vi "ini_file_read_pulse_tx.vi"(8 "error in (no error)":errorcluster, 11 "secnario config":T1={"devicess 2"=["IF_transiver_1", "IF_transiver_2"], "file paths"=[path "C:/Users/PXIe8108_Demo/Documents/CHAIM DATA/chaim/5785_sync_for_elbit/data/pdw_test_file.tdms", path "C:/Users/PXIe8108_Demo/Documents/CHAIM DATA/chaim/5785_sync_for_elbit/data/pdw_test_file.tdms", path "C:/Users/PXIe8108_Demo/Documents/CHAIM DATA/chaim/5785_sync_for_elbit/data/pdw_test_file.tdms", path "C:/Users/PXIe8108_Demo/Documents/CHAIM DATA/chaim/5785_sync_for_elbit/data/pdw_test_file.tdms"], "buffer size"=524288, "Fs  FPGA"=200000000.0, "SPC"=16.0, "center frequency (Hz) "=1000000000.0, "t clock ref"=[], "fpga rfe"=[], "tdms refs"=[], "niUsrpRio Session (out)"={"FPGA Interface"=refnum, "RIO Interface Number"=0, "Data Clock Rate"=0, "FPGA Data Clock Rate"=0, "Global Settings Register Bus"=refnum, "Radio 0 Settings Register Bus"=refnum, "Radio 1 Settings Register Bus"=refnum, "Radio Settings Bus Semaphore"=refnum, "DB Queues"=[], "Characterization Data Valid?"=FALSE, "EEPROM Header"={"Checksum"=0, "Product Code"=0, "Hardware Current Version"=0, "Hardware Oldest Compatible Version"=0, "EEPROM Map Current Version"=0, "EEPROM Map Oldest Compatible Version"=0, "User Password"="", "Pointer to Factory Header"=0, "Pointer to User Header"=0, "Recommended Interval"=0, "Number of Reserved Bytes"=9, "Number of Daughterboards"=0, "Daughterboard IDs"=[], "Daughterboard Serial Numbers"=[]}, "Device Data Header"={"Checksum"=0, "Number of Channels"=0, "Number of Gain Settings"=[], "Pointer to Characterization Data"=[], "Number of Reserved Bytes"=27, "Number of Frequencies"=[]}, "EEPROM Characterization Header"={"Checksum"=0, "Date"=timestamp(0 s since 1904-01-01), "Temperature"=0.0, "Misc. Info"="", "Pointer to Device Data Header"=0, "Number of Reserved Bytes"=28}, "Characterization Data"=[], "FPGA Current Version"=0, "FPGA Oldest Compatible Version"=0, "Fixed Logic Current Version"=0, "Fixed Logic Oldest Compatible Version"=0, "FPGA Radio Settings Bus Current Version"=0, "FPGA Radio Settings Bus Oldest Compatible Version"=0, "FPGA Board Config Current Version"=0, "FPGA Board Config Oldest Compatible Version"=0, "Daughterboard Clock Rate"=0, "daughterboard configuration session handles"=[]}, "RF gain "=10, "mode"=0, "vst_device"=[]} {"mode" scale=0.0..2.0; "RF gain" min=0 max=31 step=1; "niUsrpRio Session (out)"."Daughterboard Clock Rate" format="%#.3pHz"; "niUsrpRio Session (out)"."FPGA Data Clock Rate" format="%#.3pHz"; "niUsrpRio Session (out)"."Data Clock Rate" format="%#.3pHz"; "niUsrpRio Session (out)"."Characterization Data"."Frequencies [Hz]" format="%#_6p"; "niUsrpRio Session (out)"."EEPROM Characterization Header"."Pointer to Device Data Header" format="%x"; "niUsrpRio Session (out)"."EEPROM Characterization Header"."Checksum" format="%x"; "niUsrpRio Session (out)"."Device Data Header"."Pointer to Characterization Data" format="%x"; "niUsrpRio Session (out)"."Device Data Header"."Checksum" format="%x"; "niUsrpRio Session (out)"."EEPROM Header"."Pointer to User Header" format="%x"; "niUsrpRio Session (out)"."EEPROM Header"."Pointer to Factory Header" format="%x"; "niUsrpRio Session (out)"."EEPROM Header"."Product Code" format="%x"; "niUsrpRio Session (out)"."EEPROM Header"."Checksum" format="%x"; "center frequency (Hz)" format="%#.8p"; "buffer size" step=512}) -> (0 "error out":errorcluster, 3 "output cluster":T1={"devicess 2"=["IF_transiver_1", "IF_transiver_2"], "file paths"=[path "C:/Users/PXIe8108_Demo/Documents/CHAIM DATA/chaim/5785_sync_for_elbit/data/pdw_test_file.tdms", path "C:/Users/PXIe8108_Demo/Documents/CHAIM DATA/chaim/5785_sync_for_elbit/data/pdw_test_file.tdms", path "C:/Users/PXIe8108_Demo/Documents/CHAIM DATA/chaim/5785_sync_for_elbit/data/pdw_test_file.tdms", path "C:/Users/PXIe8108_Demo/Documents/CHAIM DATA/chaim/5785_sync_for_elbit/data/pdw_test_file.tdms"], "buffer size"=524288, "Fs  FPGA"=200000000.0, "SPC"=16.0, "center frequency (Hz) "=1000000000.0, "t clock ref"=[], "fpga rfe"=[], "tdms refs"=[], "niUsrpRio Session (out)"={"FPGA Interface"=refnum, "RIO Interface Number"=0, "Data Clock Rate"=0, "FPGA Data Clock Rate"=0, "Global Settings Register Bus"=refnum, "Radio 0 Settings Register Bus"=refnum, "Radio 1 Settings Register Bus"=refnum, "Radio Settings Bus Semaphore"=refnum, "DB Queues"=[], "Characterization Data Valid?"=FALSE, "EEPROM Header"={"Checksum"=0, "Product Code"=0, "Hardware Current Version"=0, "Hardware Oldest Compatible Version"=0, "EEPROM Map Current Version"=0, "EEPROM Map Oldest Compatible Version"=0, "User Password"="", "Pointer to Factory Header"=0, "Pointer to User Header"=0, "Recommended Interval"=0, "Number of Reserved Bytes"=9, "Number of Daughterboards"=0, "Daughterboard IDs"=[], "Daughterboard Serial Numbers"=[]}, "Device Data Header"={"Checksum"=0, "Number of Channels"=0, "Number of Gain Settings"=[], "Pointer to Characterization Data"=[], "Number of Reserved Bytes"=27, "Number of Frequencies"=[]}, "EEPROM Characterization Header"={"Checksum"=0, "Date"=timestamp(0 s since 1904-01-01), "Temperature"=0.0, "Misc. Info"="", "Pointer to Device Data Header"=0, "Number of Reserved Bytes"=28}, "Characterization Data"=[], "FPGA Current Version"=0, "FPGA Oldest Compatible Version"=0, "Fixed Logic Current Version"=0, "Fixed Logic Oldest Compatible Version"=0, "FPGA Radio Settings Bus Current Version"=0, "FPGA Radio Settings Bus Oldest Compatible Version"=0, "FPGA Board Config Current Version"=0, "FPGA Board Config Oldest Compatible Version"=0, "Daughterboard Clock Rate"=0, "daughterboard configuration session handles"=[]}, "RF gain "=10, "mode"=0, "vst_device"=[]} {"mode" scale=0.0..2.0; "RF gain" min=0 max=31 step=1; "niUsrpRio Session (out)"."Daughterboard Clock Rate" format="%#.3pHz"; "niUsrpRio Session (out)"."FPGA Data Clock Rate" format="%#.3pHz"; "niUsrpRio Session (out)"."Data Clock Rate" format="%#.3pHz"; "niUsrpRio Session (out)"."Characterization Data"."Frequencies [Hz]" format="%#_6p"; "niUsrpRio Session (out)"."EEPROM Characterization Header"."Pointer to Device Data Header" format="%x"; "niUsrpRio Session (out)"."EEPROM Characterization Header"."Checksum" format="%x"; "niUsrpRio Session (out)"."Device Data Header"."Pointer to Characterization Data" format="%x"; "niUsrpRio Session (out)"."Device Data Header"."Checksum" format="%x"; "niUsrpRio Session (out)"."EEPROM Header"."Pointer to User Header" format="%x"; "niUsrpRio Session (out)"."EEPROM Header"."Pointer to Factory Header" format="%x"; "niUsrpRio Session (out)"."EEPROM Header"."Product Code" format="%x"; "niUsrpRio Session (out)"."EEPROM Header"."Checksum" format="%x"; "center frequency (Hz)" format="%#.8p"; "buffer size" step=512})   [LabVIEW 2021]
uses:
  secnario config.ctl
  <vilib>/userdefined/High Color/nirio_resource_hc.ctl
  <instrlib>/niUsrpRio/Config/v1/Host/Public/niUsrpRio Session.ctl
  <instrlib>/_niInstr/Register Bus/v0/Host/Public/Register Bus Session.ctl
  <instrlib>/_niInstr/Register Bus/v0/Host/Private/Session Data.ctl
  <instrlib>/niUsrpRio/Config/v1/Host/Private/DB Queue Reference.ctl
  <instrlib>/niUsrpRio/Config/v1/Host/Private/Daughterboard Data.ctl
  <instrlib>/niUsrpRio/Config/v1/Host/Private/ATR state data.ctl
  <instrlib>/niUsrpRio/Config/v1/Host/Private/Antenna Configuration.ctl
  <instrlib>/niUsrpRio/Config/v1/Host/Private/CPLD Power Mode.ctl
  <instrlib>/niUsrpRio/Config/v1/Host/Public/EEPROM Header.ctl
  <instrlib>/niUsrpRio/Config/v1/Host/Public/EEPROM Device Data Header.ctl
  <instrlib>/niUsrpRio/Config/v1/Host/Public/EEPROM Characterization Header.ctl
  <instrlib>/niUsrpRio/Config/v1/Host/Public/Characterization Data.ctl
  <instrlib>/niUsrpRio/Config/v1/Host/Public/IQ Imbalance.ctl
  <instrlib>/_niInstr/Register Bus/v0/Host/niInstr Register Bus v0 Host.lvlib
  <instrlib>/niUsrpRio/Config/v1/Host/niUsrpRio Config v1 Host.lvlib
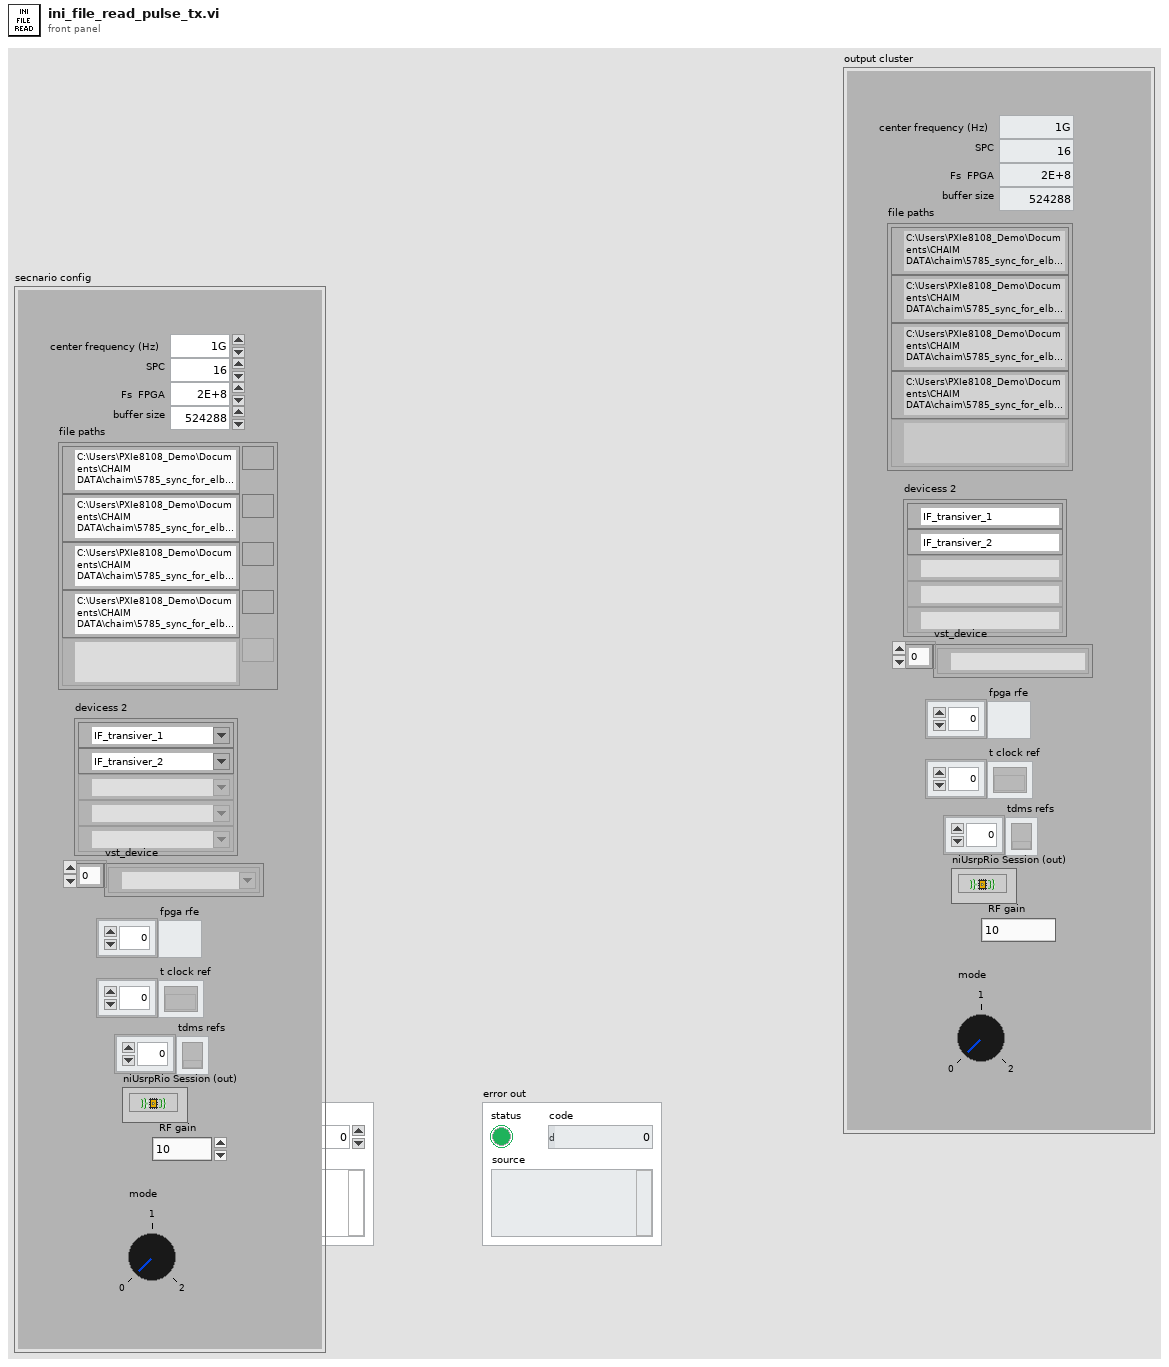
[diagram p1: front panel]
types:
  T1 = typedef "secnario config.ctl" = cluster{"devicess 2":T2[], "file paths":path[], "buffer size":u32, "Fs  FPGA":dbl, "SPC":dbl, "center frequency (Hz) ":dbl, "t clock ref":refnum<k20>[], "fpga rfe":refnum<k20>[], "tdms refs":refnum<k34>[], "niUsrpRio Session (out)":T3, "RF gain ":i32, "mode":u8, "vst_device":refnum<k15>[]}
  T2 = typedef "nirio_resource_hc.ctl" = tag
  T3 = typedef "niUsrpRio Config v1 Host.lvlib/niUsrpRio Session.ctl" = cluster{"FPGA Interface":refnum<k20>, "RIO Interface Number":u32, "Data Clock Rate":u32, "FPGA Data Clock Rate":u32, "Global Settings Register Bus":T4, "Radio 0 Settings Register Bus":T4, "Radio 1 Settings Register Bus":T4, "Radio Settings Bus Semaphore":T5, "DB Queues":T6[], "Characterization Data Valid?":bool, "EEPROM Header":T7, "Device Data Header":T8, "EEPROM Characterization Header":T9, "Characterization Data":T10[], "FPGA Current Version":u32, "FPGA Oldest Compatible Version":u32, "Fixed Logic Current Version":u32, "Fixed Logic Oldest Compatible Version":u32, "FPGA Radio Settings Bus Current Version":u32, "FPGA Radio Settings Bus Oldest Compatible Version":u32, "FPGA Board Config Current Version":u32, "FPGA Board Config Oldest Compatible Version":u32, "Daughterboard Clock Rate":u32, "daughterboard configuration session handles":u64[]}
  T4 = typedef "niInstr Register Bus v0 Host.lvlib/Register Bus Session.ctl" = refnum<queue>
  T5 = typedef "Semaphore RefNum" = refnum<k1>
  T6 = typedef "niUsrpRio Config v1 Host.lvlib/DB Queue Reference.ctl" = refnum<queue>
  T7 = typedef "niUsrpRio Config v1 Host.lvlib/EEPROM Header.ctl" = cluster{"Checksum":u32, "Product Code":u16, "Hardware Current Version":u16, "Hardware Oldest Compatible Version":u16, "EEPROM Map Current Version":u16, "EEPROM Map Oldest Compatible Version":u16, "User Password":string, "Pointer to Factory Header":u32, "Pointer to User Header":u32, "Recommended Interval":u16, "Number of Reserved Bytes":i32, "Number of Daughterboards":u8, "Daughterboard IDs":u16[], "Daughterboard Serial Numbers":string[]}
  T8 = typedef "niUsrpRio Config v1 Host.lvlib/EEPROM Device Data Header.ctl" = cluster{"Checksum":u32, "Number of Channels":u8, "Number of Gain Settings":u16[], "Pointer to Characterization Data":u32[], "Number of Reserved Bytes":i32, "Number of Frequencies":u16[]}
  T9 = typedef "niUsrpRio Config v1 Host.lvlib/EEPROM Characterization Header.ctl" = cluster{"Checksum":u32, "Date":timestamp, "Temperature":sgl, "Misc. Info":string, "Pointer to Device Data Header":u32, "Number of Reserved Bytes":i32}
  T10 = typedef "niUsrpRio Config v1 Host.lvlib/Characterization Data.ctl" = cluster{"Gains[dB]":dbl[], "Frequencies [Hz]":dbl[], "IQ Imbalance Table":T11[], "Measured Gains[dB]":dbl[][]}
  T11 = typedef "niUsrpRio Config v1 Host.lvlib/IQ Imbalance.ctl" = cluster{"Gain Imbalance [linear]":dbl, "Phase Imbalance [radians]":dbl, "Offset":cdb}
  T12 = enum16{"open", "open or create", "create or replace", "create", "open (read-only)"}
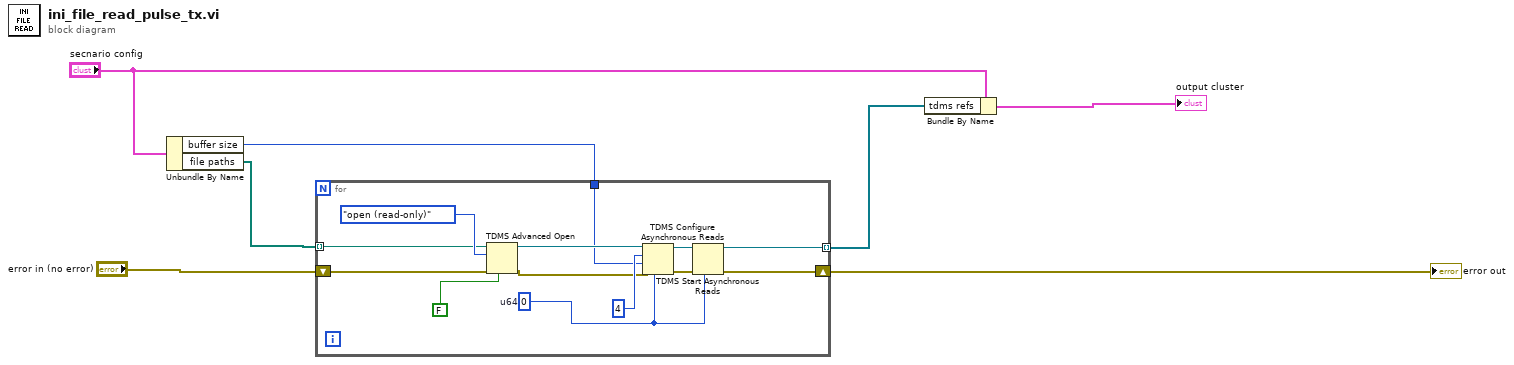
[diagram p0: block diagram]
diagram:
  n1 = Unbundle By Name("secnario config") -> ("buffer size"=w5:u32, "file paths"=w4:path[])
  n2 = for {
    tunnel: w4 -> [w18] mode=indexing
    tunnel: [w12] -> w2 mode=indexing
    shift-right: [w11] -> w6
    shift-left: "error in (no error)" -> [w10]
    tunnel: w5 -> [w8]
    w9 = u64 0  # u64
    n3 = TDMS Advanced Open(6:FALSE ("Disable Buffering? (T)"), 8:w10, 10:T12."open (read-only)" ("Operation"), 11:w18) -> (0:w13:errorcluster, 3:w14:refnum<k34>)  [unwired: 1 in, 1 out]
    n4 = TDMS Configure Asynchronous Reads(6:w9, 8:w13, 9:w8, 10:u32 4 ("Number of Buffers (4)"), 11:w14) -> (0:w16:errorcluster, 3:w17:refnum<k34>)  [unwired: 1 in]
    n5 = TDMS Start Asynchronous Reads(6:w9, 8:w16, 11:w17) -> (0:w11:errorcluster, 3:w12:refnum<k34>)  [unwired: 1 in]
  }
  "error out" <- w6
  n6 = Bundle By Name(cluster="secnario config", "tdms refs"=w2) -> (→"output cluster":T1)
